vi "magnitude_of_3d_vector.vi"(8 "error in":errorcluster, 9 "z axis component":dbl, 10 "y axis component":dbl, 11 "x axis component":dbl) -> (0 "error out":errorcluster, 3 "magnitude of 3d vector":dbl)   [LabVIEW 2017]
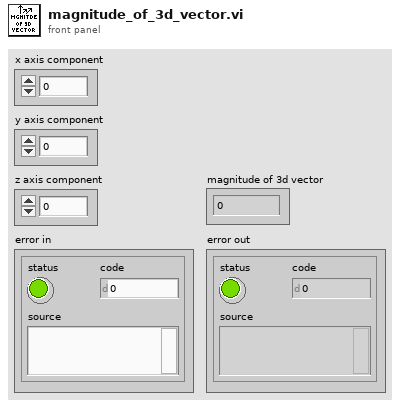
[diagram p1: front panel]
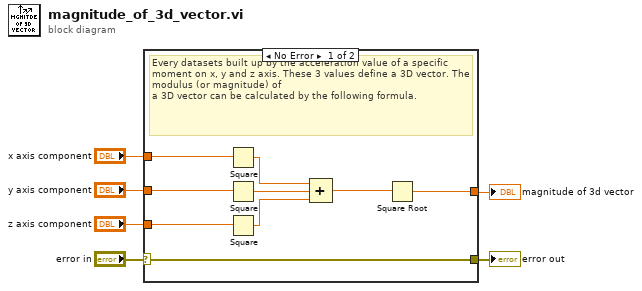
[diagram p0: block diagram]
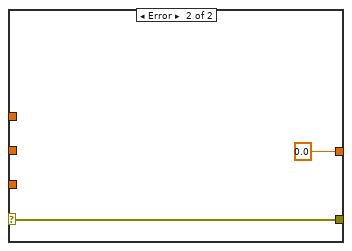
[diagram p2: hidden frame]
diagram:
  n1 = case shown="No Error" "error in" {
    selector: "error in" -> [w15 w17]
    tunnel: [w15 w17] -> w5
    tunnel: "x axis component" -> [w14 _]
    tunnel: "y axis component" -> [w13 _]
    tunnel: "z axis component" -> [w12 _]
    tunnel: [w7 0.0] -> w1
    frame No Error {
      # "Every datasets built up by the acceleration value of a specific moment on x, y and z axis. These 3 values define a 3D vector. The modulus (or magnitude) of\na 3D vector can be calculated by the following formula."
      n2 = Square(x=w14) -> (x^2=w11:dbl)
      n3 = Square(x=w13) -> (x^2=w10:dbl)
      n4 = Square(x=w12) -> (x^2=w9:dbl)
      n5 = Compound Arithmetic op=ADD(w11, w10, w9) -> (w8:dbl)
      n6 = Square Root(x=w8) -> (sqrt(x)=w7:dbl)
    }
    frame Error {
    }
  }
  "error out" <- w5
  "magnitude of 3d vector" <- w1
